vi "is missle hittting enemy.vi"(6 "Board with missles in":u32[][](array[numeric]), 9 "enemy type":dbl, 10 "colum":dbl, 11 "row":dbl) -> (3 "Boolean":bool)   [LabVIEW 2019]
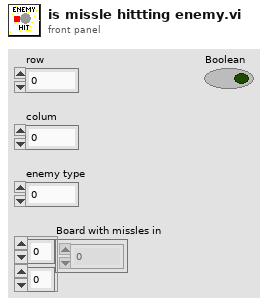
[diagram p1: front panel]
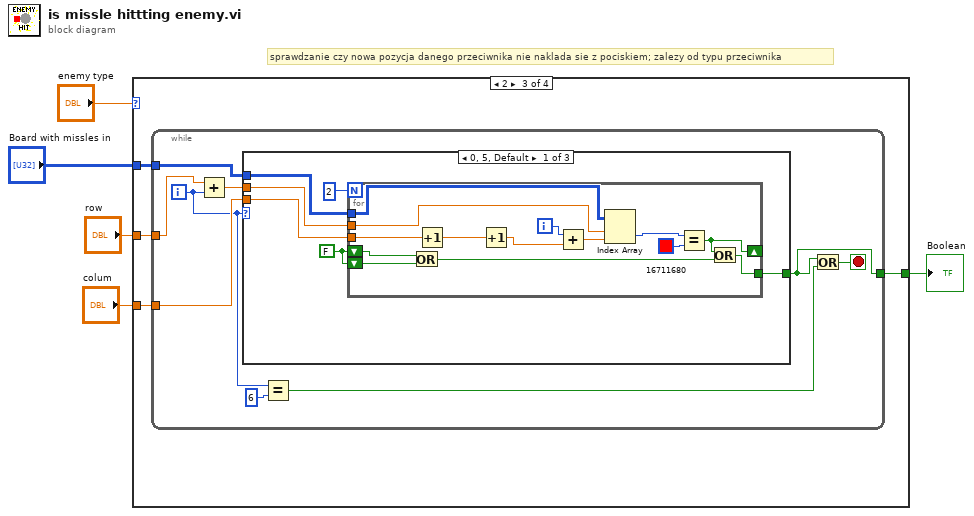
[diagram p0: block diagram]
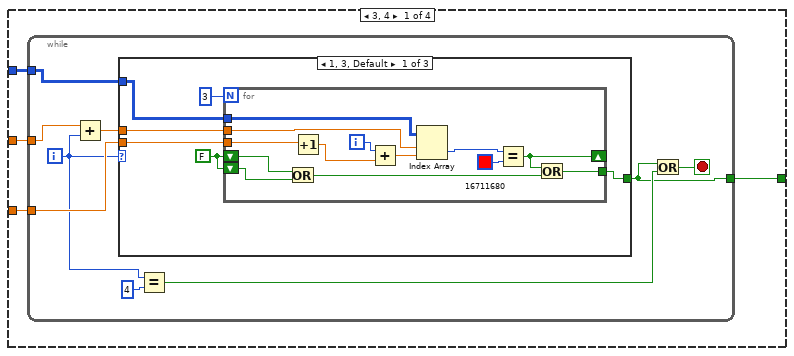
[diagram p2: hidden frame]
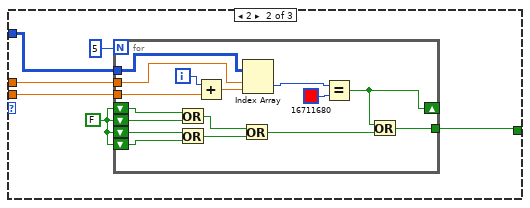
[diagram p3: hidden frame]
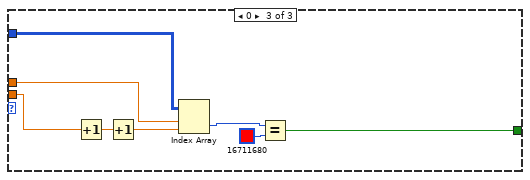
[diagram p4: hidden frame]
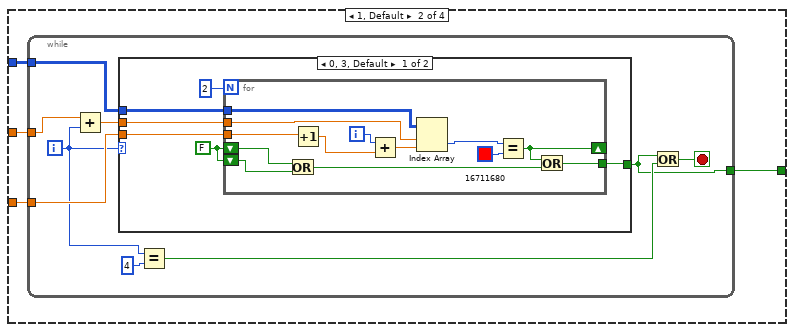
[diagram p5: hidden frame]
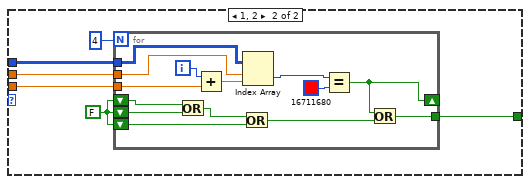
[diagram p6: hidden frame]
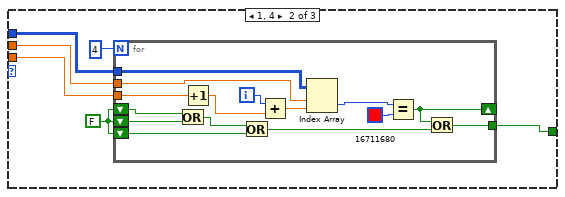
[diagram p7: hidden frame]
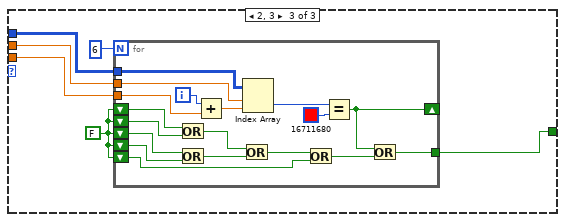
[diagram p8: hidden frame]
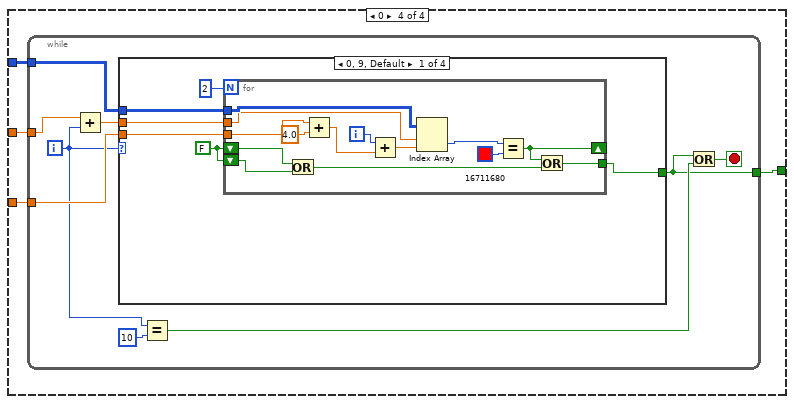
[diagram p9: hidden frame]
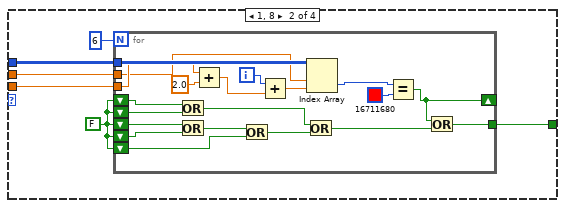
[diagram p10: hidden frame]
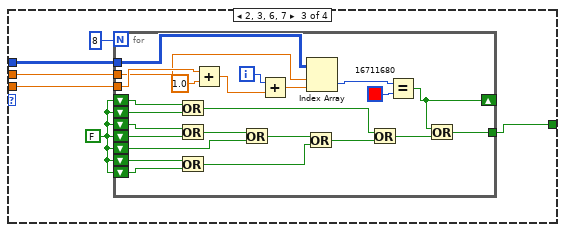
[diagram p11: hidden frame]
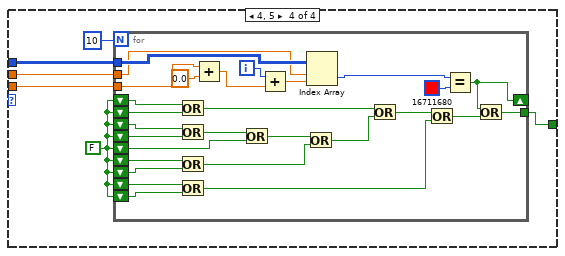
[diagram p12: hidden frame]
diagram:
  # "sprawdzanie czy nowa pozycja danego przeciwnika nie naklada sie z pociskiem; zalezy od typu przeciwnika"
  n1 = case shown="2" "enemy type" {
    tunnel: "colum" -> [w9 w71 w123 w199]
    tunnel: "row" -> [w8 w70 w122 w200]
    tunnel: "Board with missles in" -> [w7 w69 w121 w201]
    tunnel: [w6 w68 w120 w198] -> w5
    frame 3, 4 {
      n2 = while {
        tunnel: w9 -> [w18]
        tunnel: w8 -> [w13]
        tunnel: w7 -> [w17]
        tunnel: [w10] -> w6
        i -> [w12]
        stop <- w16 stop-if-true
        n3 = Add(x=w13, y=w12) -> (x+y=w11:dbl)
        n4 = case shown="1, 3, Default" w12 {
          tunnel: w18 -> [w22 w41 w61]
          tunnel: w11 -> [w23 w42 w64]
          tunnel: w17 -> [w21 w40 w67]
          tunnel: [w24 w43 w60] -> w10
          frame 1, 3, Default {
            w19 = FALSE
            n5 = for {
              N: 3 -> [_]
              tunnel: [w27] -> w24
              tunnel: w23 -> [w26]
              tunnel: w22 -> [w25]
              tunnel: w21 -> [w33]
              shift-right: [w28] -> _
              shift-left: w19 -> [w31]
              shift-left: w19 -> [w30]
              i -> [w32]
              n6 = Or(x=w31, y=w30) -> (x .or. y?=w29:bool)
              n7 = Increment(x=w25) -> (x+1=w35:dbl)
              n8 = Add(x=w32, y=w35) -> (x+y=w34:dbl)
              n9 = Index Array(array=w33, index (row)=w26, index (col)=w34) -> (element=w37:u32)
              n10 = Equal?(x=w37, y=u32 16711680) -> (x = y?=w28:bool)
              n11 = Or(x=w28, y=w29) -> (x .or. y?=w27:bool)
            }
          }
          frame 2 {
            w38 = FALSE
            n12 = for {
              N: 5 -> [_]
              tunnel: [w51] -> w43
              tunnel: w42 -> [w45]
              tunnel: w41 -> [w44]
              tunnel: w40 -> [w56]
              shift-right: [w52] -> _
              shift-left: w38 -> [w54]
              shift-left: w38 -> [w53]
              shift-left: w38 -> [w50]
              shift-left: w38 -> [w49]
              i -> [w55]
              n13 = Or(x=w54, y=w53) -> (x .or. y?=w48:bool)
              n14 = Or(x=w50, y=w49) -> (x .or. y?=w47:bool)
              n15 = Add(x=w55, y=w44) -> (x+y=w57:dbl)
              n16 = Or(x=w48, y=w47) -> (x .or. y?=w46:bool)
              n17 = Index Array(array=w56, index (row)=w45, index (col)=w57) -> (element=w59:u32)
              n18 = Equal?(x=w59, y=u32 16711680) -> (x = y?=w52:bool)
              n19 = Or(x=w52, y=w46) -> (x .or. y?=w51:bool)
            }
          }
          frame 0 {
            n20 = Increment(x=w61) -> (x+1=w63:dbl)
            n21 = Increment(x=w63) -> (x+1=w62:dbl)
            n22 = Index Array(array=w67, index (row)=w64, index (col)=w62) -> (element=w66:u32)
            n23 = Equal?(x=w66, y=u32 16711680) -> (x = y?=w60:bool)
          }
        }
        n24 = Equal?(x=w12, y=4) -> (x = y?=w14:bool)
        n25 = Or(x=w10, y=w14) -> (x .or. y?=w16:bool)
      }
    }
    frame 1, Default {
      n26 = while {
        tunnel: w71 -> [w80]
        tunnel: w70 -> [w75]
        tunnel: w69 -> [w79]
        tunnel: [w72] -> w68
        i -> [w74]
        stop <- w78 stop-if-true
        n27 = Add(x=w75, y=w74) -> (x+y=w73:dbl)
        n28 = case shown="0, 3, Default" w74 {
          tunnel: w80 -> [w84 w103]
          tunnel: w73 -> [w85 w104]
          tunnel: w79 -> [w83 w102]
          tunnel: [w86 w105] -> w72
          frame 0, 3, Default {
            w81 = FALSE
            n29 = for {
              N: 2 -> [_]
              tunnel: [w89] -> w86
              tunnel: w85 -> [w88]
              tunnel: w84 -> [w87]
              tunnel: w83 -> [w95]
              shift-right: [w90] -> _
              shift-left: w81 -> [w93]
              shift-left: w81 -> [w92]
              i -> [w94]
              n30 = Or(x=w93, y=w92) -> (x .or. y?=w91:bool)
              n31 = Increment(x=w87) -> (x+1=w97:dbl)
              n32 = Add(x=w94, y=w97) -> (x+y=w96:dbl)
              n33 = Index Array(array=w95, index (row)=w88, index (col)=w96) -> (element=w99:u32)
              n34 = Equal?(x=w99, y=u32 16711680) -> (x = y?=w90:bool)
              n35 = Or(x=w90, y=w91) -> (x .or. y?=w89:bool)
            }
          }
          frame 1, 2 {
            w100 = FALSE
            n36 = for {
              N: 4 -> [_]
              tunnel: [w112] -> w105
              tunnel: w104 -> [w107]
              tunnel: w103 -> [w106]
              tunnel: w102 -> [w116]
              shift-right: [w108] -> _
              shift-left: w100 -> [w114]
              shift-left: w100 -> [w113]
              shift-left: w100 -> [w111]
              i -> [w115]
              n37 = Or(x=w114, y=w113) -> (x .or. y?=w110:bool)
              n38 = Add(x=w115, y=w106) -> (x+y=w117:dbl)
              n39 = Or(x=w110, y=w111) -> (x .or. y?=w109:bool)
              n40 = Index Array(array=w116, index (row)=w107, index (col)=w117) -> (element=w119:u32)
              n41 = Equal?(x=w119, y=u32 16711680) -> (x = y?=w108:bool)
              n42 = Or(x=w108, y=w109) -> (x .or. y?=w112:bool)
            }
          }
        }
        n43 = Equal?(x=w74, y=4) -> (x = y?=w76:bool)
        n44 = Or(x=w72, y=w76) -> (x .or. y?=w78:bool)
      }
    }
    frame 2 {
      n45 = while {
        tunnel: w123 -> [w132]
        tunnel: w122 -> [w127]
        tunnel: w121 -> [w131]
        tunnel: [w124] -> w120
        i -> [w126]
        stop <- w130 stop-if-true
        n46 = Add(x=w127, y=w126) -> (x+y=w125:dbl)
        n47 = case shown="0, 5, Default" w126 {
          tunnel: w132 -> [w136 w156 w177]
          tunnel: w125 -> [w137 w157 w178]
          tunnel: w131 -> [w135 w155 w176]
          tunnel: [w138 w158 w179] -> w124
          frame 0, 5, Default {
            w133 = FALSE
            n48 = for {
              N: 2 -> [_]
              tunnel: [w143] -> w138
              tunnel: w137 -> [w140]
              tunnel: w136 -> [w139]
              tunnel: w135 -> [w149]
              shift-right: [w144] -> _
              shift-left: w133 -> [w147]
              shift-left: w133 -> [w146]
              i -> [w148]
              n49 = Or(x=w147, y=w146) -> (x .or. y?=w145:bool)
              n50 = Increment(x=w139) -> (x+1=w142:dbl)
              n51 = Increment(x=w142) -> (x+1=w141:dbl)
              n52 = Add(x=w148, y=w141) -> (x+y=w150:dbl)
              n53 = Index Array(array=w149, index (row)=w140, index (col)=w150) -> (element=w152:u32)
              n54 = Equal?(x=w152, y=u32 16711680) -> (x = y?=w144:bool)
              n55 = Or(x=w144, y=w145) -> (x .or. y?=w143:bool)
            }
          }
          frame 1, 4 {
            w153 = FALSE
            n56 = for {
              N: 4 -> [_]
              tunnel: [w166] -> w158
              tunnel: w157 -> [w160]
              tunnel: w156 -> [w159]
              tunnel: w155 -> [w170]
              shift-right: [w162] -> _
              shift-left: w153 -> [w168]
              shift-left: w153 -> [w167]
              shift-left: w153 -> [w165]
              i -> [w169]
              n57 = Or(x=w168, y=w167) -> (x .or. y?=w164:bool)
              n58 = Increment(x=w159) -> (x+1=w161:dbl)
              n59 = Or(x=w164, y=w165) -> (x .or. y?=w163:bool)
              n60 = Add(x=w169, y=w161) -> (x+y=w171:dbl)
              n61 = Index Array(array=w170, index (row)=w160, index (col)=w171) -> (element=w173:u32)
              n62 = Equal?(x=w173, y=u32 16711680) -> (x = y?=w162:bool)
              n63 = Or(x=w162, y=w163) -> (x .or. y?=w166:bool)
            }
          }
          frame 2, 3 {
            w174 = FALSE
            n64 = for {
              N: 6 -> [_]
              tunnel: [w192] -> w179
              tunnel: w178 -> [w181]
              tunnel: w177 -> [w180]
              tunnel: w176 -> [w194]
              shift-right: [w190] -> _
              shift-left: w174 -> [w189]
              shift-left: w174 -> [w188]
              shift-left: w174 -> [w187]
              shift-left: w174 -> [w186]
              shift-left: w174 -> [w183]
              i -> [w193]
              n65 = Or(x=w189, y=w188) -> (x .or. y?=w185:bool)
              n66 = Or(x=w187, y=w186) -> (x .or. y?=w184:bool)
              n67 = Add(x=w193, y=w180) -> (x+y=w195:dbl)
              n68 = Or(x=w185, y=w184) -> (x .or. y?=w182:bool)
              n69 = Index Array(array=w194, index (row)=w181, index (col)=w195) -> (element=w197:u32)
              n70 = Or(x=w182, y=w183) -> (x .or. y?=w191:bool)
              n71 = Equal?(x=w197, y=u32 16711680) -> (x = y?=w190:bool)
              n72 = Or(x=w190, y=w191) -> (x .or. y?=w192:bool)
            }
          }
        }
        n73 = Equal?(x=w126, y=6) -> (x = y?=w128:bool)
        n74 = Or(x=w124, y=w128) -> (x .or. y?=w130:bool)
      }
    }
    frame 0 {
      n75 = while {
        tunnel: w199 -> [w210]
        tunnel: w200 -> [w205]
        tunnel: w201 -> [w209]
        tunnel: [w202] -> w198
        i -> [w204]
        stop <- w208 stop-if-true
        n76 = Add(x=w205, y=w204) -> (x+y=w203:dbl)
        n77 = case shown="0, 9, Default" w204 {
          tunnel: w210 -> [w214 w234 w260 w290]
          tunnel: w203 -> [w215 w235 w261 w291]
          tunnel: w209 -> [w213 w233 w259 w289]
          tunnel: [w216 w236 w262 w292] -> w202
          frame 0, 9, Default {
            w211 = FALSE
            n78 = for {
              N: 2 -> [_]
              tunnel: [w221] -> w216
              tunnel: w215 -> [w217]
              tunnel: w214 -> [w218]
              tunnel: w213 -> [w227]
              shift-right: [w222] -> _
              shift-left: w211 -> [w225]
              shift-left: w211 -> [w224]
              i -> [w226]
              n79 = Or(x=w225, y=w224) -> (x .or. y?=w223:bool)
              n80 = Add(x=w218, y=4.0) -> (x+y=w220:dbl)
              n81 = Add(x=w226, y=w220) -> (x+y=w228:dbl)
              n82 = Index Array(array=w227, index (row)=w217, index (col)=w228) -> (element=w230:u32)
              n83 = Equal?(x=w230, y=u32 16711680) -> (x = y?=w222:bool)
              n84 = Or(x=w222, y=w223) -> (x .or. y?=w221:bool)
            }
          }
          frame 1, 8 {
            w231 = FALSE
            n85 = for {
              N: 6 -> [_]
              tunnel: [w248] -> w236
              tunnel: w235 -> [w244]
              tunnel: w234 -> [w245]
              tunnel: w233 -> [w253]
              shift-right: [w249] -> _
              shift-left: w231 -> [w251]
              shift-left: w231 -> [w250]
              shift-left: w231 -> [w243]
              shift-left: w231 -> [w242]
              shift-left: w231 -> [w241]
              i -> [w252]
              n86 = Or(x=w251, y=w250) -> (x .or. y?=w239:bool)
              n87 = Or(x=w243, y=w242) -> (x .or. y?=w240:bool)
              n88 = Add(x=w245, y=2.0) -> (x+y=w247:dbl)
              n89 = Or(x=w240, y=w241) -> (x .or. y?=w238:bool)
              n90 = Add(x=w252, y=w247) -> (x+y=w254:dbl)
              n91 = Or(x=w239, y=w238) -> (x .or. y?=w237:bool)
              n92 = Index Array(array=w253, index (row)=w244, index (col)=w254) -> (element=w256:u32)
              n93 = Equal?(x=w256, y=u32 16711680) -> (x = y?=w249:bool)
              n94 = Or(x=w249, y=w237) -> (x .or. y?=w248:bool)
            }
          }
          frame 2, 3, 6, 7 {
            w257 = FALSE
            n95 = for {
              N: 8 -> [_]
              tunnel: [w278] -> w262
              tunnel: w261 -> [w274]
              tunnel: w260 -> [w275]
              tunnel: w259 -> [w283]
              shift-right: [w279] -> _
              shift-left: w257 -> [w281]
              shift-left: w257 -> [w280]
              shift-left: w257 -> [w273]
              shift-left: w257 -> [w272]
              shift-left: w257 -> [w271]
              shift-left: w257 -> [w266]
              shift-left: w257 -> [w267]
              i -> [w282]
              n96 = Or(x=w281, y=w280) -> (x .or. y?=w269:bool)
              n97 = Or(x=w273, y=w272) -> (x .or. y?=w270:bool)
              n98 = Or(x=w266, y=w267) -> (x .or. y?=w264:bool)
              n99 = Add(x=w275, y=1.0) -> (x+y=w277:dbl)
              n100 = Or(x=w270, y=w271) -> (x .or. y?=w265:bool)
              n101 = Add(x=w282, y=w277) -> (x+y=w284:dbl)
              n102 = Or(x=w265, y=w264) -> (x .or. y?=w263:bool)
              n103 = Index Array(array=w283, index (row)=w274, index (col)=w284) -> (element=w286:u32)
              n104 = Or(x=w269, y=w263) -> (x .or. y?=w268:bool)
              n105 = Equal?(x=w286, y=u32 16711680) -> (x = y?=w279:bool)
              n106 = Or(x=w279, y=w268) -> (x .or. y?=w278:bool)
            }
          }
          frame 4, 5 {
            w287 = FALSE
            n107 = for {
              N: 10 -> [_]
              tunnel: [w312] -> w292
              tunnel: w291 -> [w308]
              tunnel: w290 -> [w309]
              tunnel: w289 -> [w317]
              shift-right: [w313] -> _
              shift-left: w287 -> [w315]
              shift-left: w287 -> [w314]
              shift-left: w287 -> [w307]
              shift-left: w287 -> [w306]
              shift-left: w287 -> [w305]
              shift-left: w287 -> [w301]
              shift-left: w287 -> [w302]
              shift-left: w287 -> [w297]
              shift-left: w287 -> [w296]
              i -> [w316]
              n108 = Or(x=w315, y=w314) -> (x .or. y?=w303:bool)
              n109 = Or(x=w307, y=w306) -> (x .or. y?=w304:bool)
              n110 = Or(x=w301, y=w302) -> (x .or. y?=w299:bool)
              n111 = Or(x=w297, y=w296) -> (x .or. y?=w295:bool)
              n112 = Add(x=w309, y=0.0) -> (x+y=w311:dbl)
              n113 = Or(x=w304, y=w305) -> (x .or. y?=w300:bool)
              n114 = Add(x=w316, y=w311) -> (x+y=w318:dbl)
              n115 = Or(x=w300, y=w299) -> (x .or. y?=w298:bool)
              n116 = Index Array(array=w317, index (row)=w308, index (col)=w318) -> (element=w320:u32)
              n117 = Or(x=w303, y=w298) -> (x .or. y?=w294:bool)
              n118 = Or(x=w294, y=w295) -> (x .or. y?=w293:bool)
              n119 = Equal?(x=w320, y=u32 16711680) -> (x = y?=w313:bool)
              n120 = Or(x=w313, y=w293) -> (x .or. y?=w312:bool)
            }
          }
        }
        n121 = Equal?(x=w204, y=10) -> (x = y?=w206:bool)
        n122 = Or(x=w202, y=w206) -> (x .or. y?=w208:bool)
      }
    }
  }
  "Boolean" <- w5
